vi "InTake Get.vi"() -> ()   [LabVIEW 2013]
uses:
  <vilib>/Rock Robotics/WPI/Solenoid/WPI_SolenoidValue.ctl
  InTake Global Data.vi
panel:
  in  "MoveArm":T1
  in  "TakeBall":dbl
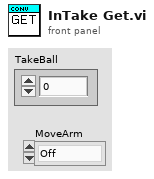
[diagram p1: front panel]
types:
  T1 = typedef "WPI_SolenoidValue.ctl" = enum16{"Off", "On", "Forward", "Reverse"}
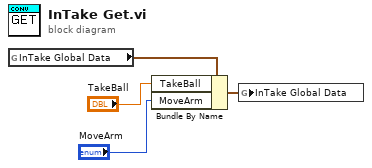
[diagram p0: block diagram]
diagram:
  n1 = global read "InTake Global Data.vi" "InTake Global Data"() -> (w2:cluster{"TakeBall":dbl, "MoveArm":T1})
  n2 = Bundle By Name(cluster=w2, "TakeBall"="TakeBall", "MoveArm"="MoveArm") -> (w1:cluster{"TakeBall":dbl, "MoveArm":T1})
  n3 = global write "InTake Global Data.vi" "InTake Global Data"(w1) -> ()
